vi "Peak_Detecting.vi"(7 "PNG output folder":path=path "C:/Users/ansom/Desktop/Agilent/PNG's From Graphs/B_BG_7to-7", 8 "Use File Offset":bool, 9 "length":i32, 10 "subset start index":i32, 11 "Folder or File":path=path "B:/SketchSET/SA03008H.20180718/08-BG_Sweep_-5to5_0.1_@0.1Hz/SA03008H.20180718.000031.itx") -> (2 "avg amplitude":dbl[](graph), 3 "avg FWHM":dbl[](graph))   [LabVIEW 2016]
uses:
  <vilib>/Analysis/baseanly.llb/Mean (DBL).vi
  <userlib>/LevyLab/LV to ITX/LVtoITX.lvclass
  <vilib>/Analysis/NI_AALBase.lvlib
panel:
  out "Waveform Graph":dbl[][](graph)
  out "x*y":dbl[][](array[numeric])
  out "peak detection locations":dbl[][](array[numeric])
  out "size(s)":i32
  out "final FWHM mean for this folder":dbl format="%p"
  out "final amplitude mean for this folder":dbl format="%p"
  out "Chopped IV":cluster{dbl[], dbl[]}(graph)
  out "Chopped dI/dV":T1(graph)
  out "input data":cluster{dbl[], dbl[]}[](graph)
  in  "Peak Threshold":dbl=1e-06 format="%p"
  in  "Diff bin size":dbl=2.0
  in  "Points to chop off the bottom edge":i32=50
  in  "Points to chop off the top edge":i32=50
  out "Iterations of loop":i32
  out "directory":bool
  out "Comments":string
  out "N__":cluster{"N1":dbl, "N2":dbl, "N3":dbl, "N4":dbl}={"N1"=0.0624995231628418, "N2"=0.0624995231628418, "N3"=0.0624995231628418, "N4"=0.0624995231628418} {"N4" format="%#_6p"; "N3" format="%#_6p"; "N2" format="%#_6p"; "N1" format="%#_6p"}
  in  "index":T2={"A"=5, "B"=3, "C"=2, "D"=0, "E"=3, "N1"=0, "N2"=0, "N3"=0, "N4"=0}
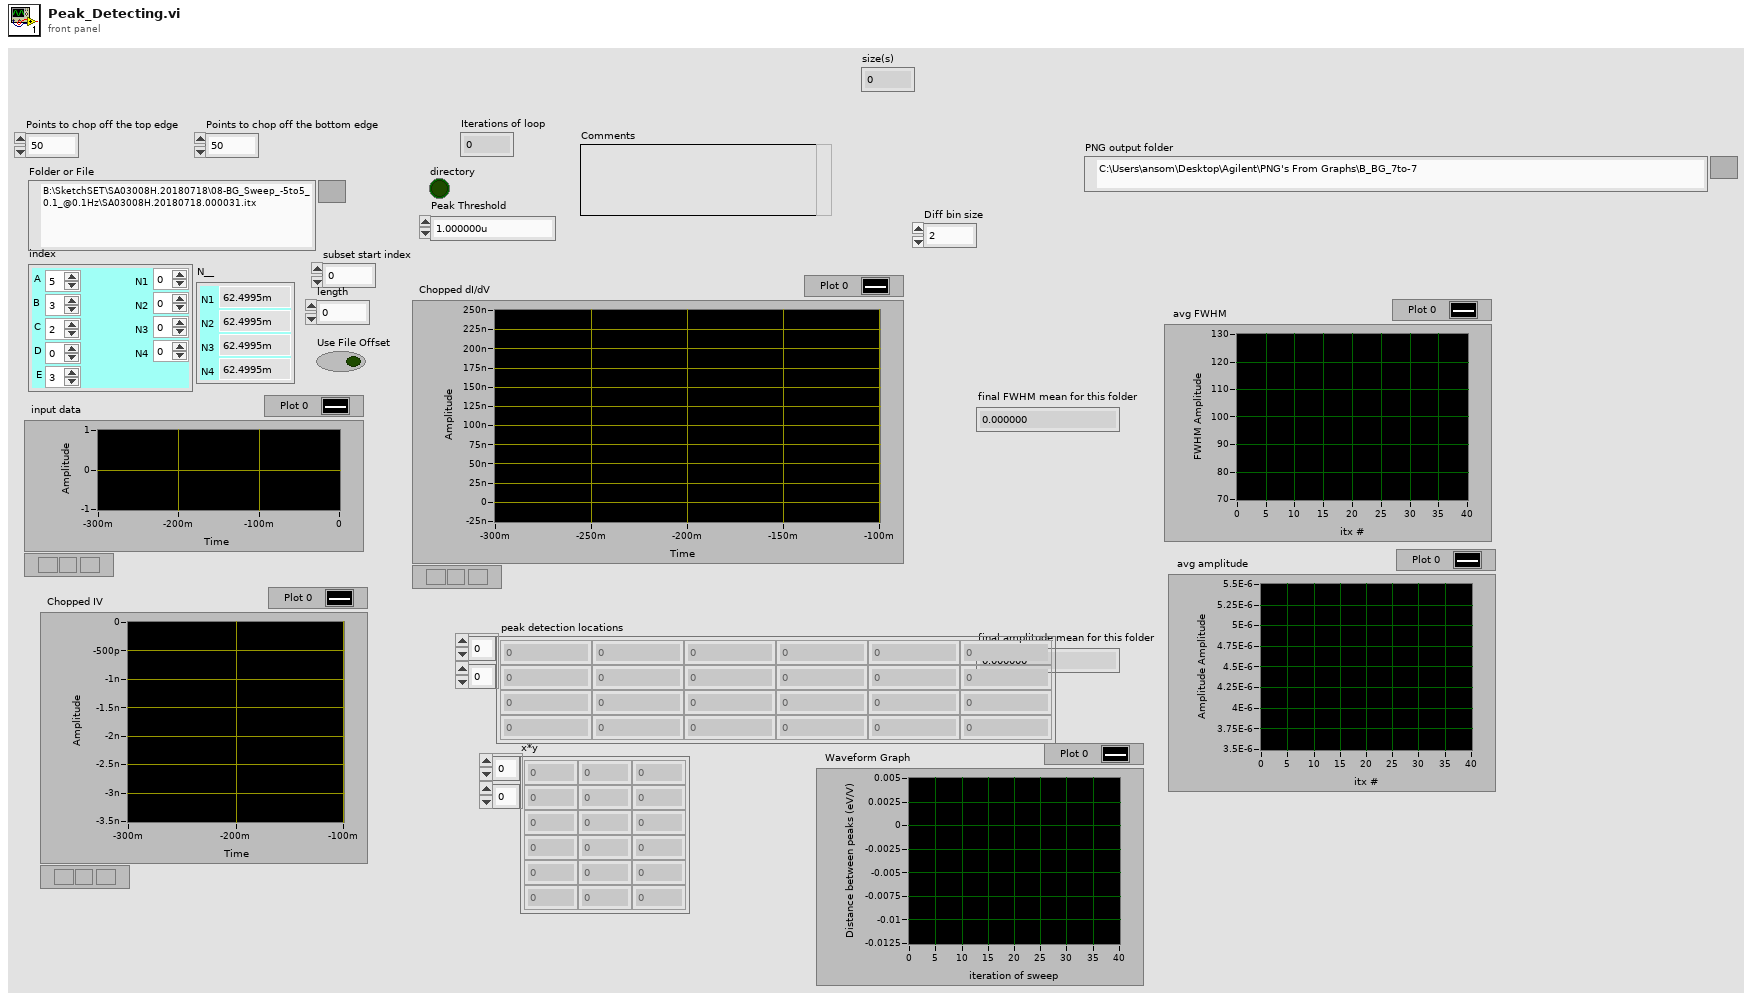
[diagram p1: front panel]
types:
  T1 = cluster{"Vsrc values":dbl[], "dI/dV values":dbl[]}
  T2 = cluster{"A":i32, "B":i32, "C":i32, "D":i32, "E":i32, "N1":i32, "N2":i32, "N3":i32, "N4":i32}
  T3 = cluster{"Decimated Array":dbl[], "Decimated Array":dbl[]}[]
  T4 = typedef "imagedata.ctl" = cluster{"image type":i32, "image depth":i32, "image":u8[], "mask":u8[], "colors":u32[], "Rectangle":cluster{"left":i16, "top":i16, "right":i16, "bottom":i16}}
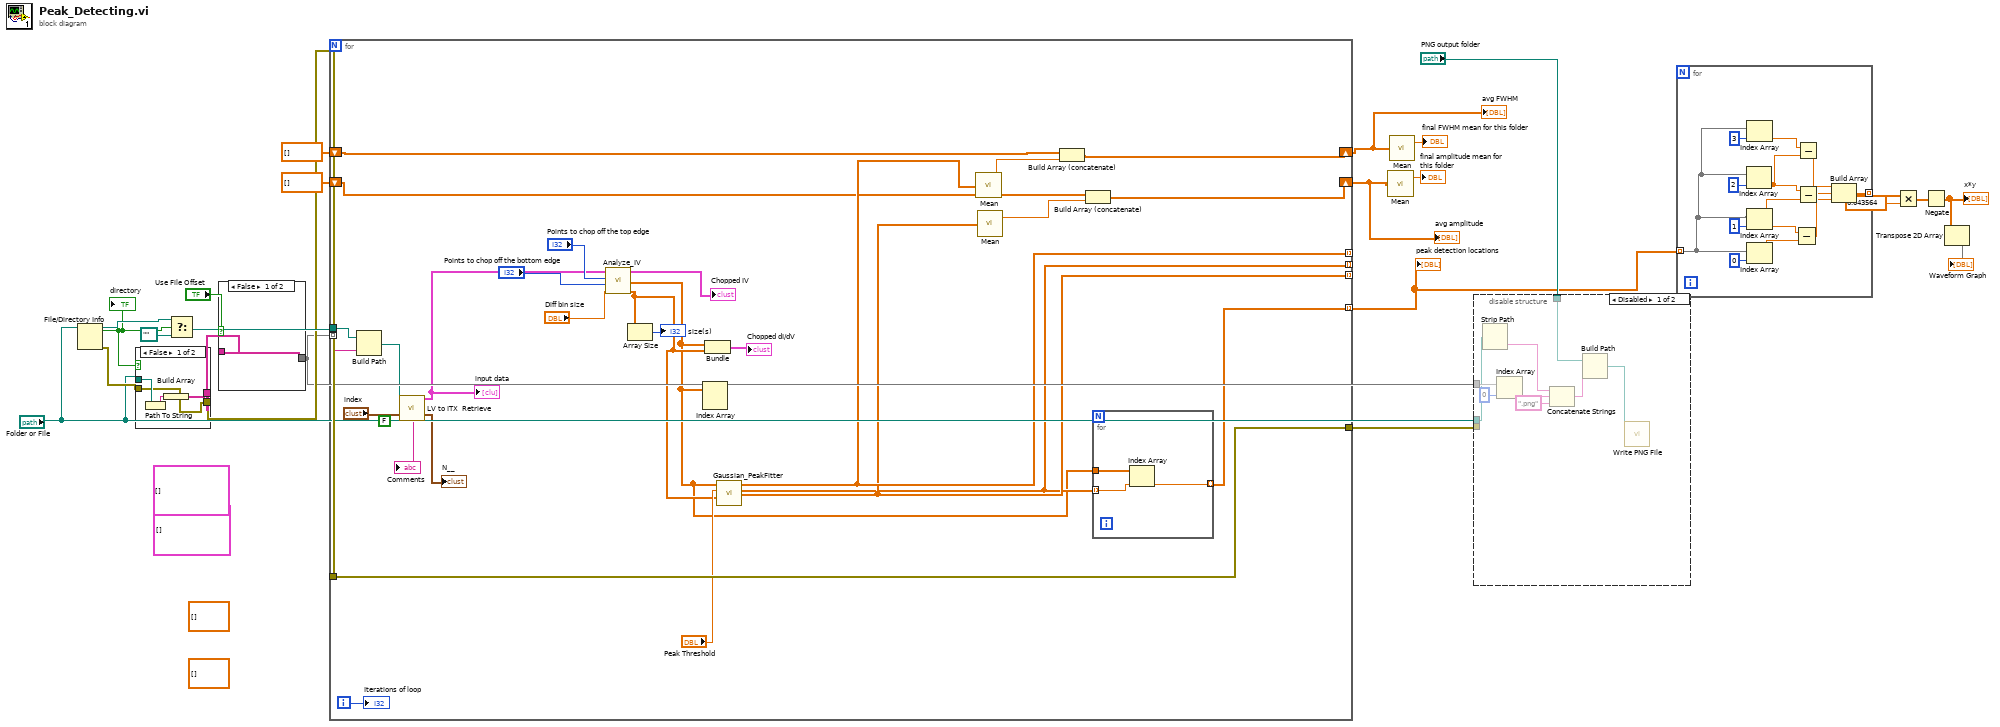
[diagram p0: block diagram]
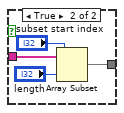
[diagram p3: hidden frame]
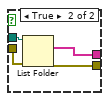
[diagram p4: hidden frame]
diagram:
  (unwired) dbl[][] []
  (unwired) dbl[][] []
  (unwired) T3 []
  (unwired) cluster{dbl[], dbl[]}[] []
  n1 = File/Directory Info(path="Folder or File") -> (path out=w23:path, directory=w22:bool, error out=w24:errorcluster)  [unwired: 1 in, 4 out]
  "directory" <- w22
  n2 = case shown="False" w22 {
    tunnel: "Folder or File" -> [w28 w32]
    tunnel: w24 -> [w25 w31]
    tunnel: [w26 w30] -> w19
    tunnel: [w25 w29] -> w18
    frame False {
      n3 = Path To String(path=w28) -> (string=w27:string)
      n4 = Build Array(w27) -> (w26:string[])
    }
    frame True {
      n5 = List Folder(path=w32, error in=w31) -> (filenames=w30:string[], error out=w29:errorcluster)  [unwired: 2 in, 2 out]
    }
  }
  n6 = Select(t=w23, s=w22, f=path "") -> (s? t:f=w21:path)
  n7 = case shown="False" "Use File Offset" {
    tunnel: w19 -> [w33 w37]
    tunnel: [w33 w36] -> w17
    frame False {
    }
    frame True {
      n8 = Array Subset(array=w37, index="subset start index", length="length") -> (w36:string[])
    }
  }
  n9 = for {
    tunnel: w17 -> [w62] mode=indexing
    tunnel: w21 -> [w60]
    tunnel: [w58] -> w15
    tunnel: w18 -> [w58]
    shift-right: [w48] -> w8
    shift-left: dbl[] [] -> [w46]
    shift-right: [w43] -> w9
    shift-left: dbl[] [] -> [w45]
    tunnel: [w50] -> _ mode=indexing
    tunnel: [w49] -> _ mode=indexing
    tunnel: [w41] -> _ mode=indexing
    tunnel: [w39] -> w6 mode=indexing
    i -> [w59]
    (unwired) FALSE ("stop")
    n10 = Build Path(base path=w60, name or relative path=w62) -> (appended path=w61:path)
    n11 = call <userlib>:"LV to ITX  Retrieve.vi"("File or Folder Path"=w61, "index"="index") -> ("A vs B"=w53:cluster{dbl[], dbl[]}[], "N"=→"N__":cluster{"N1":dbl, "N2":dbl, "N3":dbl, "N4":dbl}, "Comments"=→"Comments":string)  [unwired: 9 in, 2 out]
    "input data" <- w53
    n12 = call "Analyze_IV.vi"("Diff bin size"="Diff bin size", "Points to chop off the bottom edge"="Points to chop off the bottom edge", "Points to chop off the top edge"="Points to chop off the top edge", "A vs B IN"=w53) -> ("dI/dV values"=w40:dbl[], "Vsrc values"=w38:dbl[], "IV curve subsection"=→"Chopped IV":cluster{dbl[], dbl[]})  [unwired: 4 in, 1 out]
    n13 = Array Size(array=w40) -> (size(s)=→"size(s)":i32)
    n14 = Index Array(array=w38) -> ()  [unwired: 2 in, 2 out]
    n15 = Bundle("Vsrc values"=w38, "dI/dV values"=w40) -> (→"Chopped dI/dV":T1)  [unwired: 1 in]
    n16 = call "Gaussian_PeakFitter.vi"("Y array in"=w40, "Peak Threshold"="Peak Threshold", "X array in"=w38) -> ("Amplitudes"=w49:dbl[], "peak detection locations"=w41:dbl[], "FWHM"=w50:dbl[])  [unwired: 6 in]
    n17 = call-poly <vilib>:"Mean.vi"("X"=w50) -> ("mean"=w47:dbl)  [unwired: 1 out]
    n18 = call-poly <vilib>:"Mean.vi"("X"=w49) -> ("mean"=w44:dbl)  [unwired: 1 out]
    n19 = Build Array (concatenate)(w46, w47) -> (w48:dbl[])
    n20 = Build Array (concatenate)(w45, w44) -> (w43:dbl[])
    n21 = for {
      tunnel: w41 -> [w68] mode=indexing
      tunnel: w38 -> [w67]
      tunnel: [w66] -> w39 mode=indexing
      n22 = Index Array(array=w67, index=w68) -> (element=w66:dbl)
    }
    "Iterations of loop" <- w59
  }
  "avg amplitude" <- w9
  "avg FWHM" <- w8
  "peak detection locations" <- w6
  n23 = call-poly <vilib>:"Mean.vi"("X"=w9) -> ("mean"=→"final amplitude mean for this folder":dbl)  [unwired: 1 out]
  n24 = call-poly <vilib>:"Mean.vi"("X"=w8) -> ("mean"=→"final FWHM mean for this folder":dbl)  [unwired: 1 out]
  n25 = disable-structure shown="Disabled" {
    disable-tunnel: w17 -> [w80 _]
    disable-tunnel: "PNG output folder" -> [w78 _]
    disable-tunnel: w15 -> [w76 _]
    disable-tunnel: "Folder or File" -> [w69 _]
    frame Disabled {
      n26 = Strip Path(path=w69) -> (name=w70:string)  [unwired: 1 out]
      n27 = Index Array(array=w80, index=0) -> (element=w73:string)
      n28 = Concatenate Strings(w70, w73, ".png" ("string")) -> (w72:string)
      n29 = Build Path(base path=w78, name or relative path=w72) -> (appended path=w79:path)
      n30 = call <vilib>:"Write PNG File.vi"("path to PNG file"=w79) -> ("error in (no error)"=w74:errorcluster, "image data"=w75:T4)  [unwired: 7 in, 2 out]
    }
    frame Enabled {
    }
  }
  n31 = for {
    tunnel: w6 -> [w92] mode=indexing
    tunnel: [w84] -> w4 mode=indexing
    n32 = Index Array(array=w92, index=2) -> (element=w86:dbl)
    n33 = Index Array(array=w92, index=3) -> (element=w87:dbl)
    n34 = Index Array(array=w92, index=1) -> (element=w85:dbl)
    n35 = Index Array(array=w92, index=0) -> (element=w93:dbl)
    n36 = Subtract(x=w85, y=w93) -> (x-y=w83:dbl)
    n37 = Subtract(x=w87, y=w86) -> (x-y=w82:dbl)
    n38 = Subtract(x=w86, y=w85) -> (x-y=w81:dbl)
    n39 = Build Array(w83, w81, w82) -> (w84:dbl[])
  }
  n40 = Multiply(x=w4, y=0.043564) -> (x*y=w3:dbl[][])
  n41 = Negate(x=w3) -> (-x=w2:dbl[][])
  "x*y" <- w2
  n42 = Transpose 2D Array(2D array=w2) -> (transposed array=→"Waveform Graph":dbl[][])
